vi "Shutdown Python Connector.vi"(7 "Server Alias":string, 8 "error in (no error)":errorcluster) -> (0 "error out":errorcluster)   [LabVIEW 2013, in "TS.lvlib"]
doc: "This VI tells the Python side to quit."
uses:
  TS.lvlib
  LabVIEW Python Connector Message.ctl
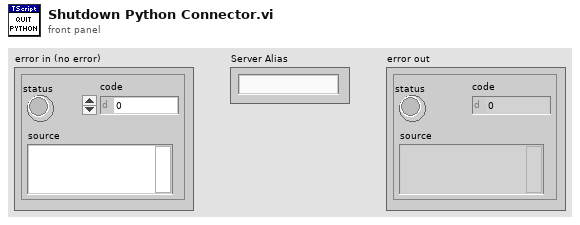
[diagram p1: front panel]
types:
  T1 = typedef "TS.lvlib/LabVIEW Python Connector Message.ctl" = cluster{"Command":string, "Data":string[], "Script ID":i64, "LabVIEW Server ID":string, "Python Message ID":i32}
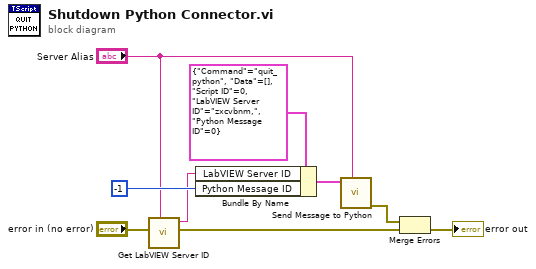
[diagram p0: block diagram]
diagram:
  n1 = call "Get LabVIEW Server ID.vi"("Server Alias"="Server Alias", "Error In"="error in (no error)") -> ("Error Out"=w3:errorcluster, "LabVIEW Server ID"=w2:string)  [unwired: 8 in]
  n2 = Bundle By Name(cluster=T1 {"Command"="quit_python", "Data"=[], "Script ID"=0, "LabVIEW Server ID"="zxcvbnm,", "Python Message ID"=0} ("Message"), "LabVIEW Server ID"=w2, "Python Message ID"=-1) -> (w4:T1)
  n3 = call "Send Message to Python.vi"("Server Alias"="Server Alias", "Message"=w4) -> ("error out"=w7:errorcluster)  [unwired: 9 in]
  n4 = Merge Errors(w7, w3) -> (→"error out":errorcluster)
